vi "EnergyLevelsDynamic.vi"(9 "Z-Position":dbl, 10 "Up/Down Control":bool=TRUE) -> (1 "Energy Level":picture)   [LabVIEW 2023]
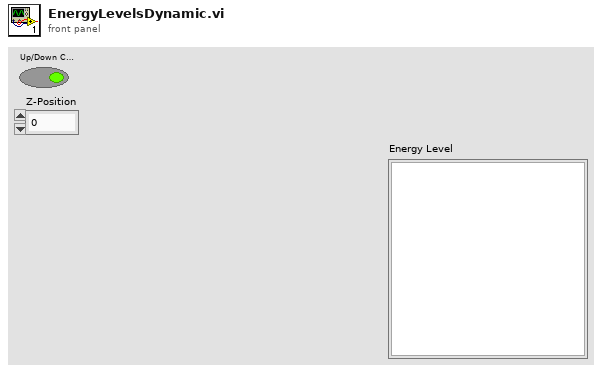
[diagram p1: front panel]
types:
  T1 = cluster{cluster{i32, i32}, cluster{i32, i32}, cluster{i32, i32}, cluster{i32, i32}}
  T2 = cluster{cluster{"lower limit":dbl, "upper limit":dbl}, cluster{"lower limit":dbl, "upper limit":dbl}}
  T3 = cluster{cluster{"lower limit":dbl, "upper limit":dbl}, cluster{dbl, "upper limit":dbl}, cluster{dbl, "upper limit":dbl}, cluster{"lower limit":dbl, "upper limit":dbl}}
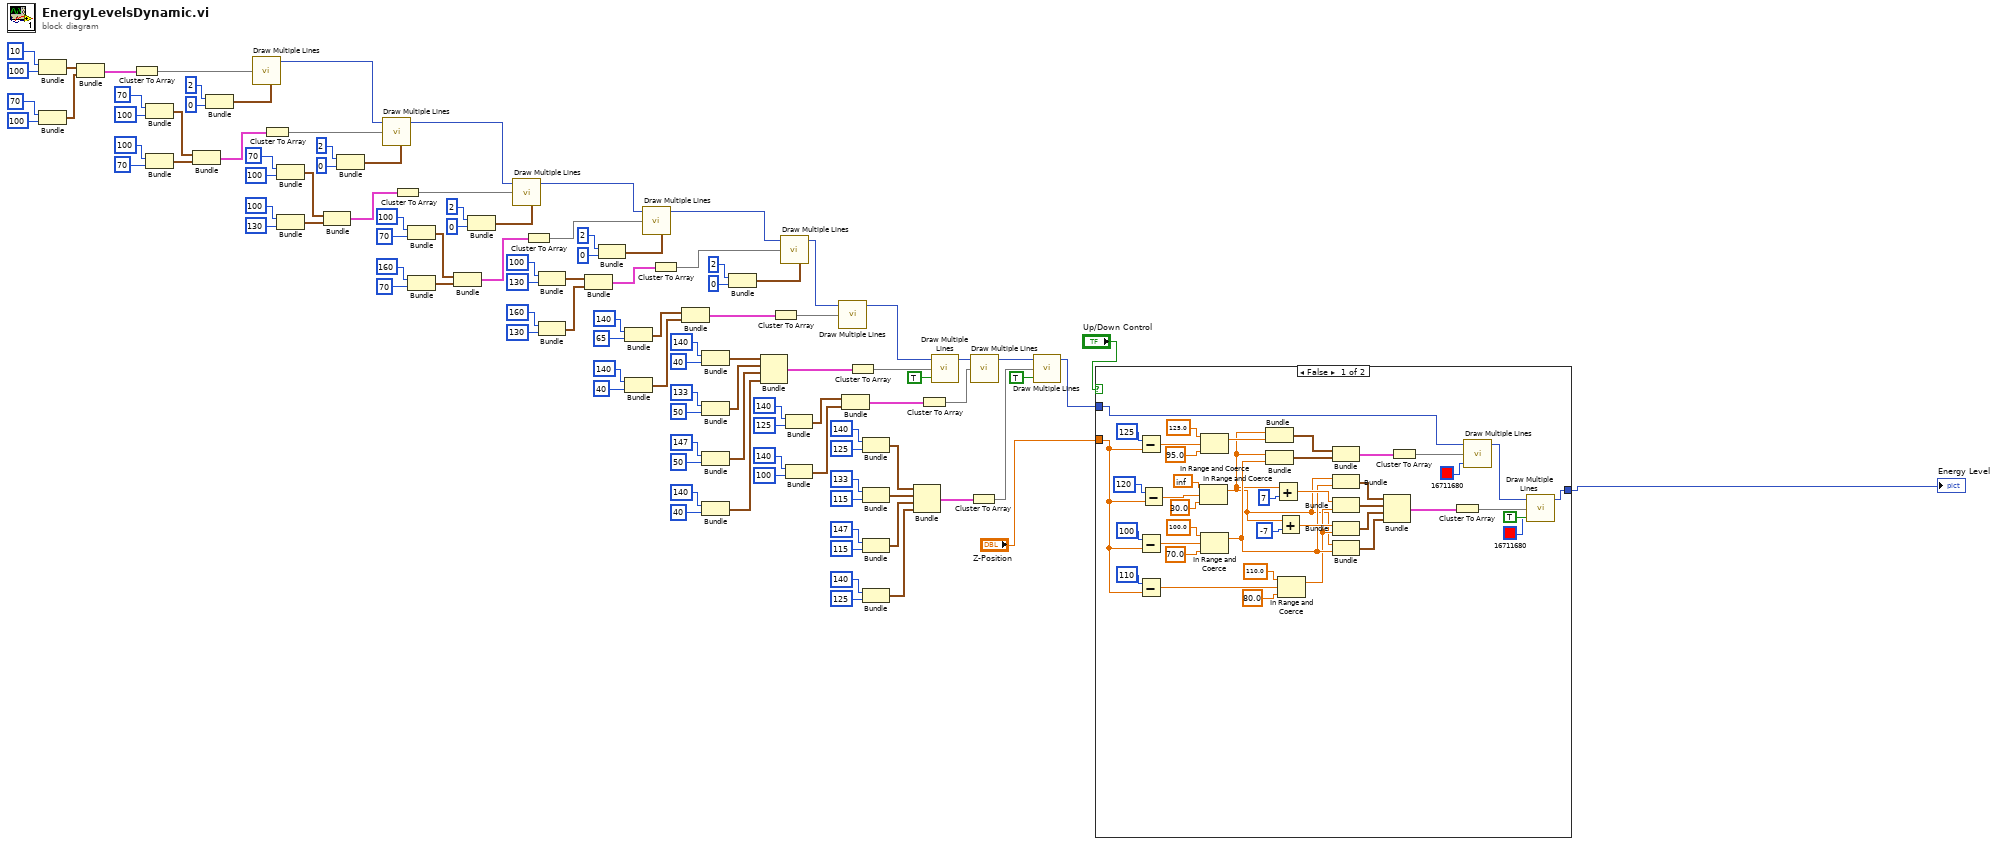
[diagram p0: block diagram]
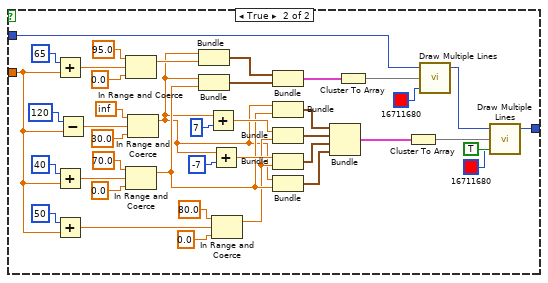
[diagram p2: hidden frame]
diagram:
  n1 = Bundle(10, 100) -> (w113:cluster{i32, i32})  [unwired: 1 in]
  n2 = Bundle(70, 100) -> (w112:cluster{i32, i32})  [unwired: 1 in]
  n3 = Bundle(w113, w112) -> (w106:cluster{cluster{i32, i32}, cluster{i32, i32}})  [unwired: 1 in]
  n4 = Cluster To Array(cluster=w106) -> (array=w107:cluster{i32, i32}[])
  n5 = Bundle(70, 100) -> (w102:cluster{i32, i32})  [unwired: 1 in]
  n6 = Bundle(100, 70) -> (w101:cluster{i32, i32})  [unwired: 1 in]
  n7 = Bundle(w102, w101) -> (w99:cluster{cluster{i32, i32}, cluster{i32, i32}})  [unwired: 1 in]
  n8 = Bundle(2, 0) -> (w105:cluster{i32, i32})  [unwired: 1 in]
  n9 = call <vilib>:"Draw Multiple Lines.vi"("line endpoints"=w107, "pen"=w105) -> ("new picture"=w96:picture)  [unwired: 7 in]
  n10 = Cluster To Array(cluster=w99) -> (array=w100:cluster{i32, i32}[])
  n11 = Bundle(70, 100) -> (w90:cluster{i32, i32})  [unwired: 1 in]
  n12 = Bundle(100, 130) -> (w89:cluster{i32, i32})  [unwired: 1 in]
  n13 = Bundle(w90, w89) -> (w87:cluster{cluster{i32, i32}, cluster{i32, i32}})  [unwired: 1 in]
  n14 = Bundle(2, 0) -> (w95:cluster{i32, i32})  [unwired: 1 in]
  n15 = call <vilib>:"Draw Multiple Lines.vi"("picture"=w96, "line endpoints"=w100, "pen"=w95) -> ("new picture"=w79:picture)  [unwired: 6 in]
  n16 = Cluster To Array(cluster=w87) -> (array=w88:cluster{i32, i32}[])
  n17 = Bundle(100, 70) -> (w78:cluster{i32, i32})  [unwired: 1 in]
  n18 = Bundle(160, 70) -> (w77:cluster{i32, i32})  [unwired: 1 in]
  n19 = Bundle(w78, w77) -> (w75:cluster{cluster{i32, i32}, cluster{i32, i32}})  [unwired: 1 in]
  n20 = Bundle(2, 0) -> (w84:cluster{i32, i32})  [unwired: 1 in]
  n21 = call <vilib>:"Draw Multiple Lines.vi"("picture"=w79, "line endpoints"=w88, "pen"=w84) -> ("new picture"=w67:picture)  [unwired: 6 in]
  n22 = Cluster To Array(cluster=w75) -> (array=w76:cluster{i32, i32}[])
  n23 = Bundle(100, 130) -> (w66:cluster{i32, i32})  [unwired: 1 in]
  n24 = Bundle(160, 130) -> (w65:cluster{i32, i32})  [unwired: 1 in]
  n25 = Bundle(w66, w65) -> (w63:cluster{cluster{i32, i32}, cluster{i32, i32}})  [unwired: 1 in]
  n26 = Bundle(2, 0) -> (w72:cluster{i32, i32})  [unwired: 1 in]
  n27 = Bundle(140, 65) -> (w51:cluster{i32, i32})  [unwired: 1 in]
  n28 = Bundle(140, 40) -> (w52:cluster{i32, i32})  [unwired: 1 in]
  n29 = call <vilib>:"Draw Multiple Lines.vi"("picture"=w67, "line endpoints"=w76, "pen"=w72) -> ("new picture"=w55:picture)  [unwired: 6 in]
  n30 = Cluster To Array(cluster=w63) -> (array=w64:cluster{i32, i32}[])
  n31 = Bundle(w51, w52) -> (w53:cluster{cluster{i32, i32}, cluster{i32, i32}})  [unwired: 1 in]
  n32 = Bundle(140, 40) -> (w46:cluster{i32, i32})  [unwired: 1 in]
  n33 = Bundle(133, 50) -> (w42:cluster{i32, i32})  [unwired: 1 in]
  n34 = Bundle(147, 50) -> (w39:cluster{i32, i32})  [unwired: 1 in]
  n35 = Bundle(140, 40) -> (w34:cluster{i32, i32})  [unwired: 1 in]
  n36 = Bundle(2, 0) -> (w60:cluster{i32, i32})  [unwired: 1 in]
  n37 = Bundle(w46, w42, w39, w34) -> (w32:T1)  [unwired: 1 in]
  n38 = Cluster To Array(cluster=w53) -> (array=w54:cluster{i32, i32}[])
  n39 = call <vilib>:"Draw Multiple Lines.vi"("picture"=w55, "line endpoints"=w64, "pen"=w60) -> ("new picture"=w5:picture)  [unwired: 6 in]
  n40 = Bundle(140, 125) -> (w12:cluster{i32, i32})  [unwired: 1 in]
  n41 = Bundle(140, 100) -> (w13:cluster{i32, i32})  [unwired: 1 in]
  n42 = call <vilib>:"Draw Multiple Lines.vi"("picture"=w5, "line endpoints"=w54) -> ("new picture"=w31:picture)  [unwired: 7 in]
  n43 = Bundle(w12, w13) -> (w14:cluster{cluster{i32, i32}, cluster{i32, i32}})  [unwired: 1 in]
  n44 = Cluster To Array(cluster=w32) -> (array=w45:cluster{i32, i32}[])
  n45 = Bundle(140, 125) -> (w30:cluster{i32, i32})  [unwired: 1 in]
  n46 = Bundle(133, 115) -> (w26:cluster{i32, i32})  [unwired: 1 in]
  n47 = Bundle(147, 115) -> (w23:cluster{i32, i32})  [unwired: 1 in]
  n48 = Bundle(140, 125) -> (w18:cluster{i32, i32})  [unwired: 1 in]
  n49 = Bundle(w30, w26, w23, w18) -> (w16:T1)  [unwired: 1 in]
  n50 = Cluster To Array(cluster=w14) -> (array=w15:cluster{i32, i32}[])
  n51 = call <vilib>:"Draw Multiple Lines.vi"("picture"=w31, "line endpoints"=w45, "fill?(F)"=TRUE) -> ("new picture"=w7:picture)  [unwired: 6 in]
  n52 = Cluster To Array(cluster=w16) -> (array=w29:cluster{i32, i32}[])
  n53 = call <vilib>:"Draw Multiple Lines.vi"("picture"=w7, "line endpoints"=w15) -> ("new picture"=w6:picture)  [unwired: 7 in]
  n54 = call <vilib>:"Draw Multiple Lines.vi"("picture"=w6, "line endpoints"=w29, "fill?(F)"=TRUE) -> ("new picture"=w4:picture)  [unwired: 6 in]
  n55 = case shown="False" "Up/Down Control" {
    tunnel: w4 -> [w115 w182]
    tunnel: [w116 w181] -> w3
    tunnel: "Z-Position" -> [w114 w159]
    frame False {
      n56 = Subtract(x=125, y=w114) -> (x-y=w131:dbl)
      n57 = Subtract(x=100, y=w114) -> (x-y=w127:dbl)
      n58 = Subtract(x=110, y=w114) -> (x-y=w121:dbl)
      n59 = Subtract(x=120, y=w114) -> (x-y=w119:dbl)
      n60 = In Range and Coerce(upper limit=inf, x=w119, lower limit=30.0) -> (coerced(x)=w120:dbl)  [unwired: 1 out]
      n61 = In Range and Coerce(upper limit=125.0, x=w131, lower limit=95.0) -> (coerced(x)=w130:dbl)  [unwired: 1 out]
      n62 = In Range and Coerce(upper limit=100.0, x=w127, lower limit=70.0) -> (coerced(x)=w126:dbl)  [unwired: 1 out]
      n63 = Bundle("lower limit"=w120, "upper limit"=w130) -> (w147:cluster{"lower limit":dbl, "upper limit":dbl})  [unwired: 1 in]
      n64 = Bundle("lower limit"=w120, "upper limit"=w126) -> (w146:cluster{"lower limit":dbl, "upper limit":dbl})  [unwired: 1 in]
      n65 = Add(x=w120, y=7) -> (x+y=w139:dbl)
      n66 = Add(x=w120, y=-7) -> (x+y=w137:dbl)
      n67 = In Range and Coerce(upper limit=110.0, x=w121, lower limit=80.0) -> (coerced(x)=w123:dbl)  [unwired: 1 out]
      n68 = Bundle(w147, w146) -> (w136:T2)  [unwired: 1 in]
      n69 = Bundle("lower limit"=w120, "upper limit"=w126) -> (w154:cluster{"lower limit":dbl, "upper limit":dbl})  [unwired: 1 in]
      n70 = Bundle(w139, "upper limit"=w123) -> (w152:cluster{dbl, "upper limit":dbl})  [unwired: 1 in]
      n71 = Bundle(w137, "upper limit"=w123) -> (w151:cluster{dbl, "upper limit":dbl})  [unwired: 1 in]
      n72 = Bundle("lower limit"=w120, "upper limit"=w126) -> (w150:cluster{"lower limit":dbl, "upper limit":dbl})  [unwired: 1 in]
      n73 = Bundle(w154, w152, w151, w150) -> (w148:T3)  [unwired: 1 in]
      n74 = Cluster To Array(cluster=w136) -> (array=w145:cluster{"lower limit":dbl, "upper limit":dbl}[])
      n75 = Cluster To Array(cluster=w148) -> (array=w153:cluster{"lower limit":dbl, "upper limit":dbl}[])
      n76 = call <vilib>:"Draw Multiple Lines.vi"("picture"=w115, "line endpoints"=w145, "color(black)"=u32 16711680) -> ("new picture"=w144:picture)  [unwired: 6 in]
      n77 = call <vilib>:"Draw Multiple Lines.vi"("picture"=w144, "line endpoints"=w153, "fill?(F)"=TRUE, "color(black)"=u32 16711680) -> ("new picture"=w116:picture)  [unwired: 5 in]
    }
    frame True {
      n78 = Add(x=65, y=w159) -> (x+y=w170:dbl)
      n79 = Add(x=40, y=w159) -> (x+y=w166:dbl)
      n80 = Add(x=50, y=w159) -> (x+y=w160:dbl)
      n81 = Subtract(x=120, y=w159) -> (x-y=w157:dbl)
      n82 = In Range and Coerce(upper limit=95.0, x=w170, lower limit=0.0) -> (coerced(x)=w169:dbl)  [unwired: 1 out]
      n83 = In Range and Coerce(upper limit=70.0, x=w166, lower limit=0.0) -> (coerced(x)=w165:dbl)  [unwired: 1 out]
      n84 = In Range and Coerce(upper limit=inf, x=w157, lower limit=30.0) -> (coerced(x)=w158:dbl)  [unwired: 1 out]
      n85 = Bundle("lower limit"=w158, "upper limit"=w169) -> (w188:cluster{"lower limit":dbl, "upper limit":dbl})  [unwired: 1 in]
      n86 = Bundle("lower limit"=w158, "upper limit"=w165) -> (w187:cluster{"lower limit":dbl, "upper limit":dbl})  [unwired: 1 in]
      n87 = Add(x=w158, y=7) -> (x+y=w178:dbl)
      n88 = Add(x=w158, y=-7) -> (x+y=w176:dbl)
      n89 = In Range and Coerce(upper limit=80.0, x=w160, lower limit=0.0) -> (coerced(x)=w162:dbl)  [unwired: 1 out]
      n90 = Bundle(w188, w187) -> (w175:T2)  [unwired: 1 in]
      n91 = Bundle("lower limit"=w158, "upper limit"=w165) -> (w195:cluster{"lower limit":dbl, "upper limit":dbl})  [unwired: 1 in]
      n92 = Bundle(w178, "upper limit"=w162) -> (w193:cluster{dbl, "upper limit":dbl})  [unwired: 1 in]
      n93 = Bundle(w176, "upper limit"=w162) -> (w192:cluster{dbl, "upper limit":dbl})  [unwired: 1 in]
      n94 = Bundle("lower limit"=w158, "upper limit"=w165) -> (w191:cluster{"lower limit":dbl, "upper limit":dbl})  [unwired: 1 in]
      n95 = Bundle(w195, w193, w192, w191) -> (w189:T3)  [unwired: 1 in]
      n96 = Cluster To Array(cluster=w175) -> (array=w186:cluster{"lower limit":dbl, "upper limit":dbl}[])
      n97 = Cluster To Array(cluster=w189) -> (array=w194:cluster{"lower limit":dbl, "upper limit":dbl}[])
      n98 = call <vilib>:"Draw Multiple Lines.vi"("picture"=w182, "line endpoints"=w186, "color(black)"=u32 16711680) -> ("new picture"=w185:picture)  [unwired: 6 in]
      n99 = call <vilib>:"Draw Multiple Lines.vi"("picture"=w185, "line endpoints"=w194, "fill?(F)"=TRUE, "color(black)"=u32 16711680) -> ("new picture"=w181:picture)  [unwired: 5 in]
    }
  }
  "Energy Level" <- w3
